vi "设置字体.vi"(8 "error in (no error)":errorcluster caption="错误输入（无错误）", 11 "程序响应 输入":refnum<class "程序响应.lvclass">) -> (0 "error out":errorcluster caption="错误输出", 3 "程序响应 输出":refnum<class "程序响应.lvclass">)   [LabVIEW 2018, in "程序响应.lvlib" / "程序响应.lvclass"]
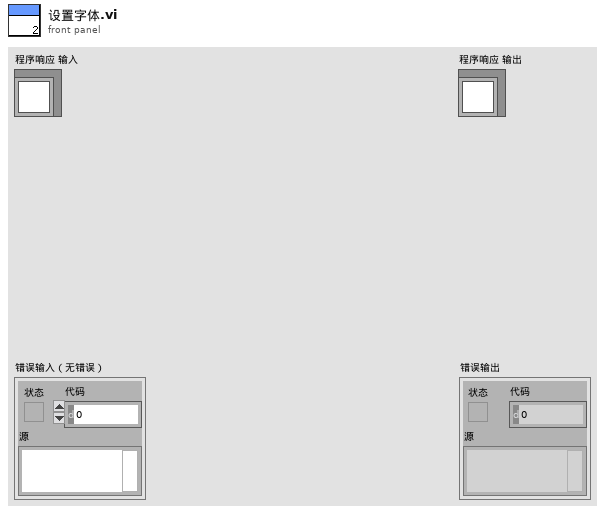
[diagram p1: front panel]
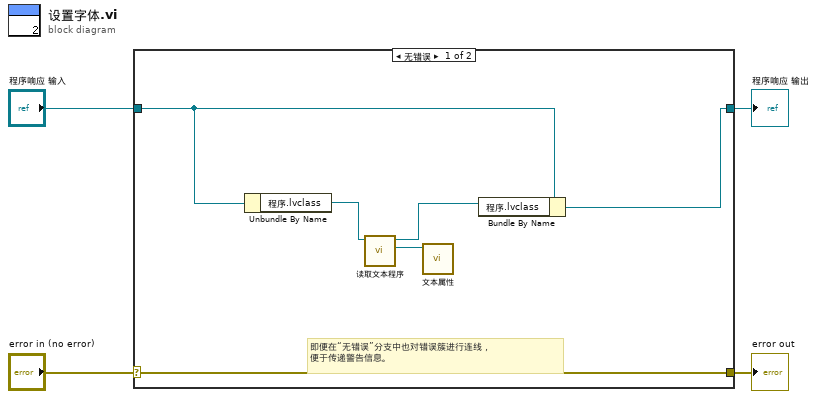
[diagram p0: block diagram]
diagram:
  n1 = case shown="无错误" "error in (no error)" {
    selector: "error in (no error)" -> [w10 w12]
    tunnel: [w10 w12] -> w3
    tunnel: [w8 w11] -> w1
    tunnel: "程序响应 输入" -> [w9 w11]
    frame No Error {
      # "即便在“无错误”分支中也对错误簇进行连线，\n便于传递警告信息。"
      n2 = Unbundle By Name(w9) -> ("程序.lvclass"=w7:refnum<class "程序.lvclass">)
      n3 = call-dynamic "读取文本程序.vi"("程序输入"=w7) -> ("文本程序"=w6:refnum<vi>, "程序输出"=w5:refnum<class "程序.lvclass">)  [unwired: 8 in, 1 out]
      n4 = call "文本属性.vi"("引用"=w6) -> ()  [unwired: 11 in]
      n5 = Bundle By Name(cluster=w9, "程序.lvclass"=w5) -> (w8:refnum<class "程序响应.lvclass">)
    }
    frame Error {
    }
  }
  "error out" <- w3
  "程序响应 输出" <- w1
